vi "Uruchomienie.vi"() -> ()   [LabVIEW 2015]
uses:
  Typedefs/Analiza.ctl
  Typedefs/dane.ctl
  Typedefs/mqttinputs.ctl
  Libraries/MQTT.lvlibp
panel:
  in  "Cisnienie 2":T1 {"P" format="%#.1f"}
  in  "SKSVdial":T2 {"SV" format="%#.1f"; "SK" format="%#.1f"}
  out "value":i32 format="%.0b"
  in  "Start":bool
  out "Zapisane":bool
  in  "Do Bazy":bool
  out "Opis":string
  out "Tacho":dbl format="%#.0f"
  out "Moc Zamowiona":dbl
  out "Typ Palnika":string
  out "Typ Wymiennika":string
  out "SNW":string
  out "SNP":string
  out "cisnienieOK":bool
  in  "Cisnienie":bool
  in  "Analiza":T3 {"I" format="%#.0f"; "CO2" format="%#.1f"; "CO" format="%#.0f"; "O2" format="%#.1f"}
  out "SKSVOK":bool
  in  "SKSV":bool
  out "AnalizaMinKlientOK":bool
  out "AnalizaMaxKlientOK":bool
  out "AnalizaMinOK":bool
  out "AnalizaMaxOK":bool
  in  "AnalizaMinKlient":bool
  in  "AnalizaMaxKlient":bool
  in  "AnalizaMin":bool
  in  "AnalizaMax":bool
  in  "BtnMaxLufa":bool
  in  "BtnMin":bool
  in  "PWMMin":dbl=15.0
  in  "BtnMax Klient":bool
  in  "PWM Max Klient":dbl=90.0
  in  "Kas":bool
  out "Awaria":bool
  out "PWM":dbl
  in  "BtnMax":bool
  in  "PWM Max":dbl=100.0
  in  "BtnMin Klient":bool
  in  "PWMMinKlient":dbl=15.0
  in  "BtnStart":bool
  out "MOC":dbl format="%#_1g"
  in  "Uruchamia:":u16(ring) items=["------", "RADZIWON TOMASZ", "RADZIWON MICHAŁ", "HARBANOWICZ FRANCISZEK", "JANUSZKIEWICZ JAKUB", "PIOTROWSKI DAMIAN", "WISZNIEWSKI JERZY", "BOHM ŁUKASZ"]
  in  "Temat":u16(ring) items=["------", "197-B", "2534-A"]
  in  "PWMStart":dbl=25.0
  in  "Nawiew_f":dbl=7.0
  in  "Nawiew":bool
  out "GAZ":bool
  in  "Zaplon":bool
  # "Hz"
  # "kW"
  # "21-24: 25%\npozostale 45%"
  # "%"
  # "%"
  # "Hz"
  # "%"
  # "%"
  # "%"
  # "%"
  # "Pa"
  # "mm"
  # "mm"
  # "Pmax 4%-5%\nPmin 3%-6.5%"
  # "%"
  # "%"
  # "ppm"
  # "<100ppm"
  # "uA"
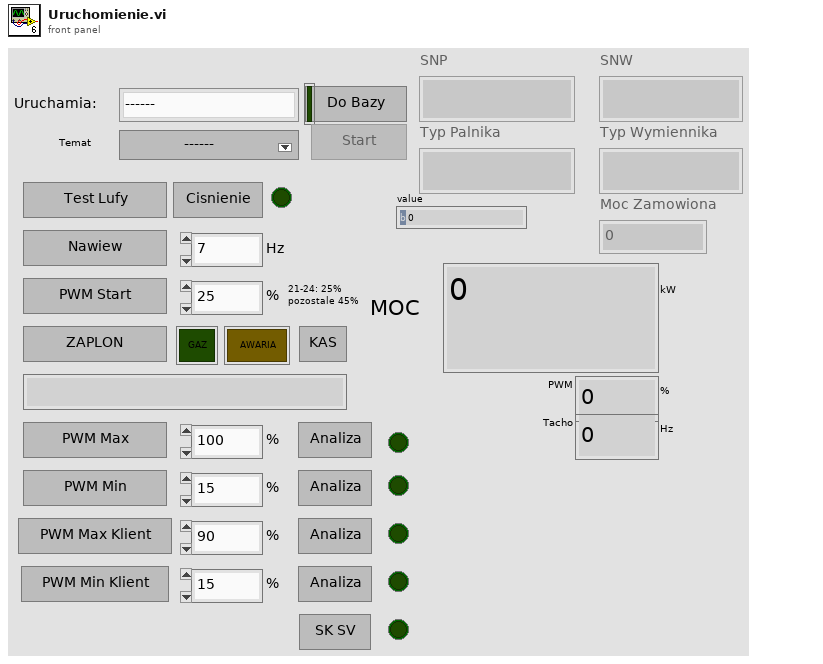
[diagram p1: front panel]
types:
  T1 = cluster{"P":dbl, "OK Button":bool, "Cancel Button":bool}
  T2 = cluster{"SK":dbl, "OK Button":bool, "Cancel Button":bool, "SV":dbl}
  T3 = typedef "Analiza.ctl" = cluster{"O2":dbl, "CO":dbl, "OK Button":bool, "Cancel Button":bool, "CO2":dbl, "I":dbl}
  T4 = typedef "MQTT.lvlibp/Broadcast Events--cluster.ctl" = cluster{"Module Did Init":refnum<user-event>, "Status Updated":refnum<user-event>, "Error Reported":refnum<user-event>, "Module Did Stop":refnum<user-event>, "Update Module Execution Status":refnum<user-event>, "Message":refnum<user-event>}
  T5 = enum8{"Enabled", "Disabled", "Disabled and Grayed Out"}
  T6 = enum32{"invalid app kind", "Development System", "Run Time System", "Student Edition", "Embedded LabVIEW", "Evaluation", "Custom"}
  T7 = typedef "dane.ctl" = cluster{"P":cluster{"max":dbl, "min":dbl, "klientmax":dbl, "klientmin":dbl}, "CO":cluster{"max":dbl, "min":dbl, "klientmax":dbl, "klientmin":dbl}, "CO2":cluster{"max":dbl, "min":dbl, "klientmax":dbl, "klientmin":dbl}, "O2":cluster{"max":dbl, "min":dbl, "klientmax":dbl, "klientmin":dbl}, "I":cluster{"max":dbl, "min":dbl, "klientmax":dbl, "klientmin":dbl}, "n":cluster{"max":dbl, "min":dbl, "klientmax":dbl, "klientmin":dbl}, "pwm":cluster{"klientmax":dbl, "klientmin":dbl}, "valve":cluster{"SK":dbl, "SV":dbl}, "pLufa100":dbl, "data":cluster{"Uruchomil":dbl, "Temat":string, "Podtemat":string, "Uwagi":string}}
  T8 = enum32{"Invalid", "Standard", "Closed", "Hidden", "Minimized", "Maximized"}
  T9 = typedef "mqttinputs.ctl" = cluster{"Power":dbl, "PWM":i32, "Tacho":i32, "Gaz":bool, "Awaria":bool, "dP":dbl, "Praca":bool, "DKG":bool}
  T10 = cluster{refnum<vi>[], "Core":cluster{"Current VI Reference":refnum<vi>, "Close Panel on Exit?":bool}, "controls":refnum<vi>[], "Kto-Lista":string[], "Kto-Lista-Num":i32[], "Kto":u8, "Tematy-Lista":string[], "TematyDane":string[][], "Temat":string, "Data":T7, "PWM":cluster{" start":i32, "min":i32, "max":i32, "moc":i32, "min klient":i32, "max klient":i32}, "CurrentPWM":i32, "broadcasts":variant, "Subscriptions":variant, "Inputs":T9, "Analiza":string}
  T11 = cluster{" start":i32, "min":i32, "max":i32, "moc":i32, "min klient":i32, "max klient":i32}
  T12 = cluster{"Current VI Reference":refnum<vi>, "Close Panel on Exit?":bool}
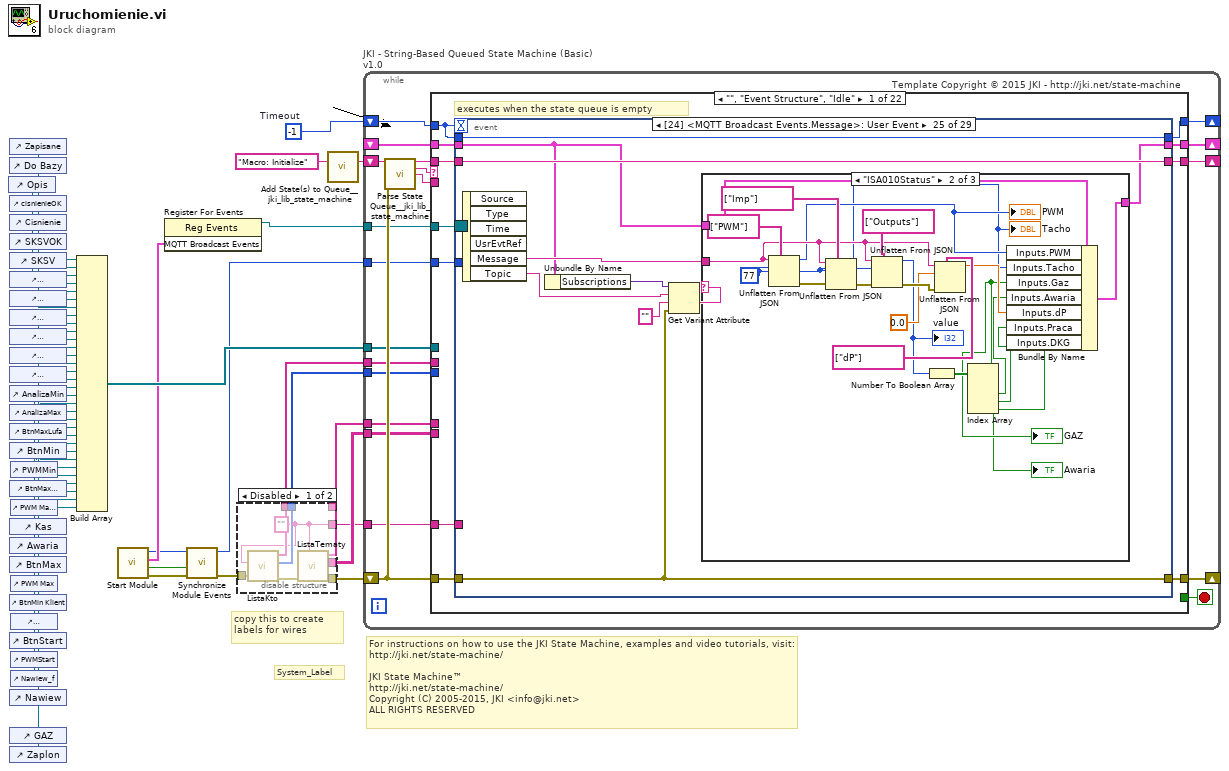
[diagram p0: block diagram]
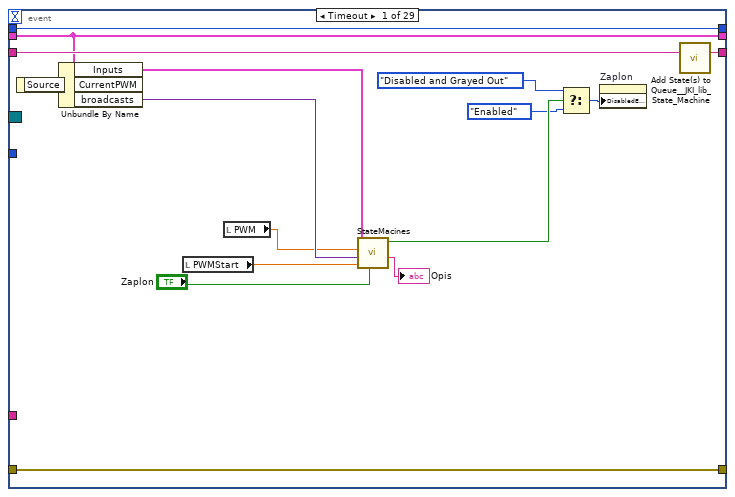
[diagram p3: hidden frame]
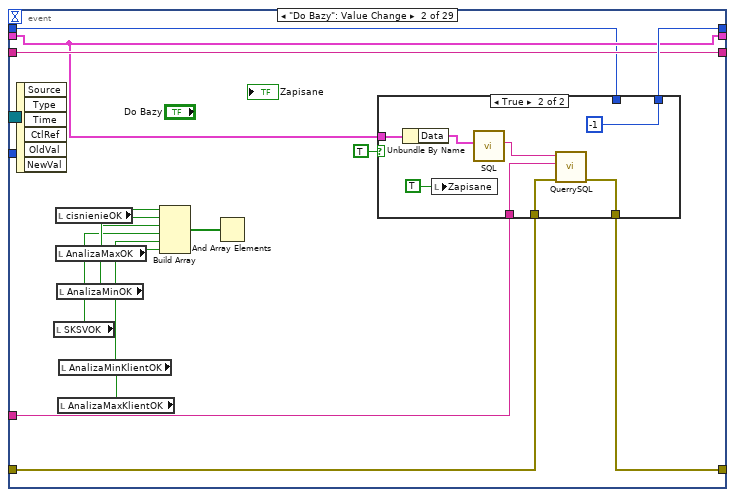
[diagram p4: hidden frame]
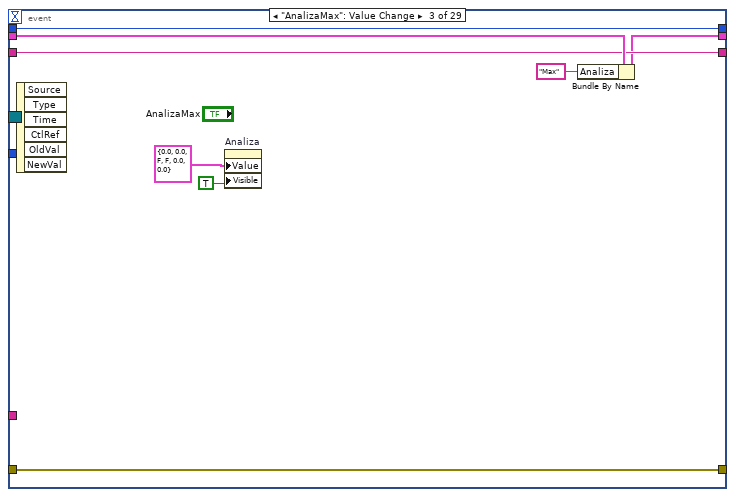
[diagram p6: hidden frame]
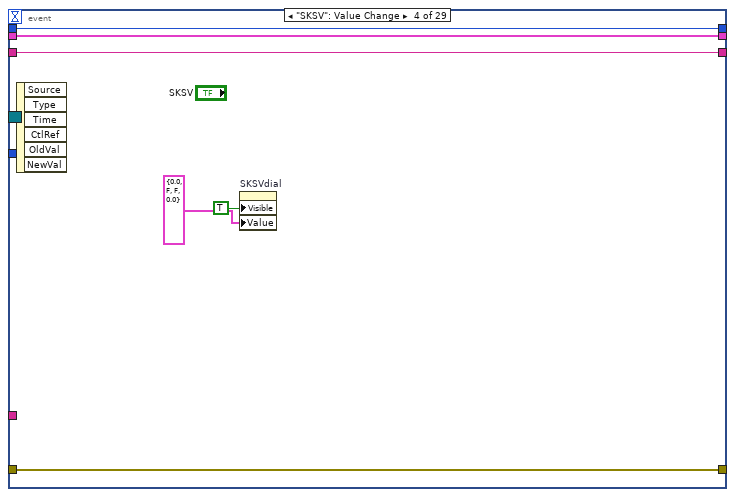
[diagram p7: hidden frame]
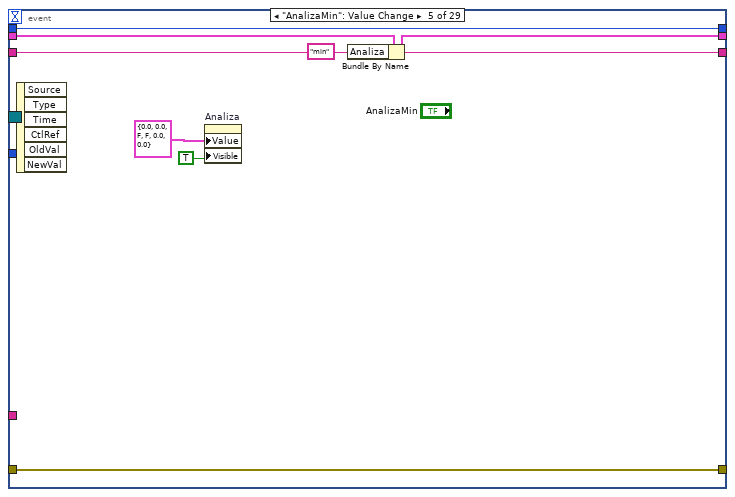
[diagram p8: hidden frame]
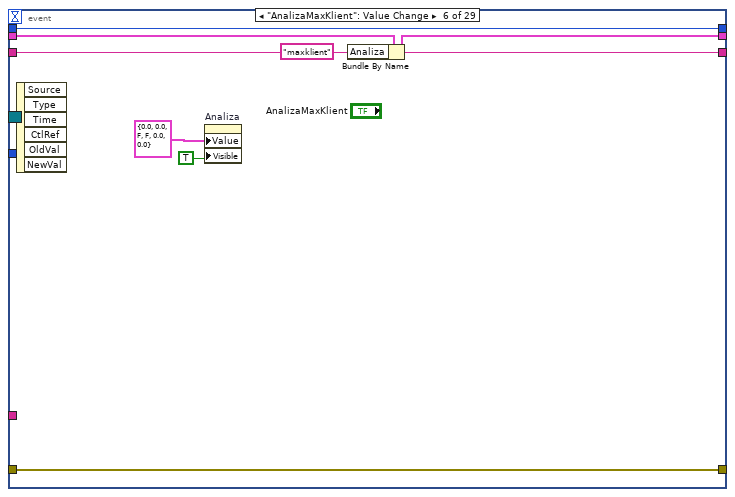
[diagram p9: hidden frame]
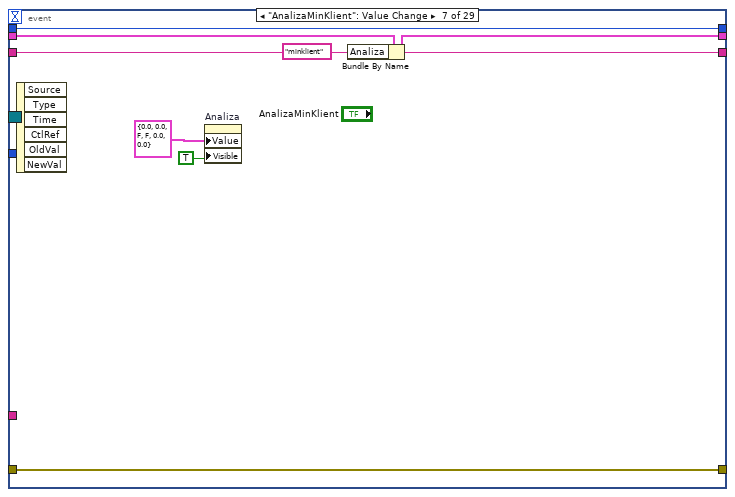
[diagram p10: hidden frame]
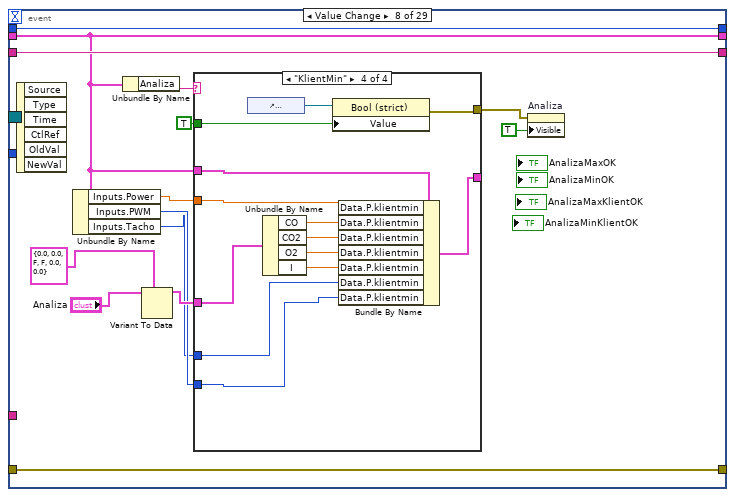
[diagram p11: hidden frame]
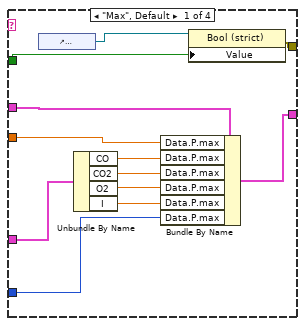
[diagram p12: hidden frame]
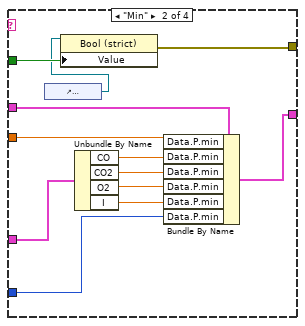
[diagram p13: hidden frame]
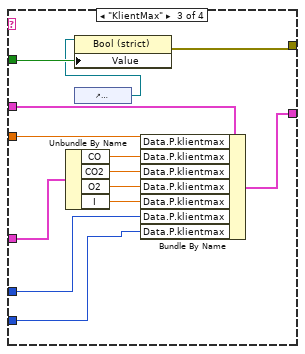
[diagram p14: hidden frame]
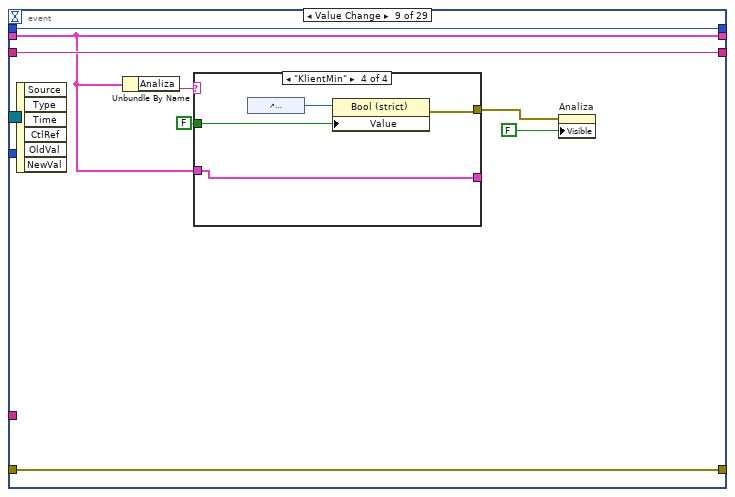
[diagram p15: hidden frame]
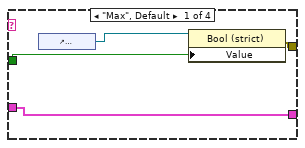
[diagram p16: hidden frame]
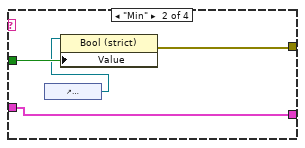
[diagram p17: hidden frame]
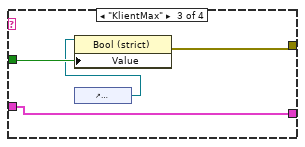
[diagram p18: hidden frame]
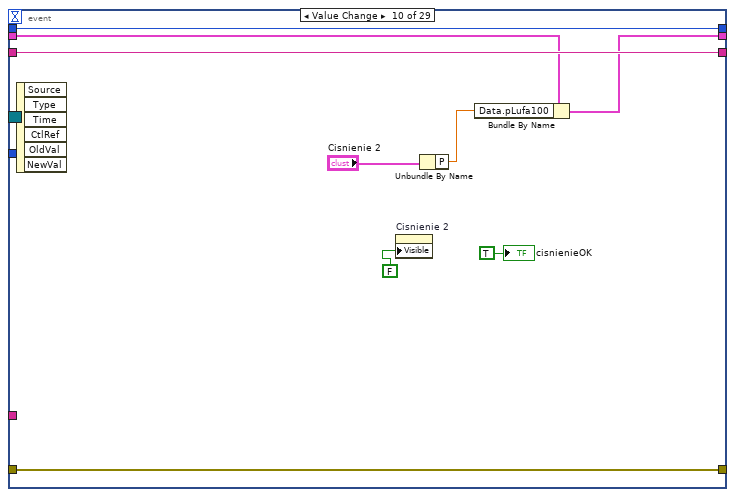
[diagram p19: hidden frame]
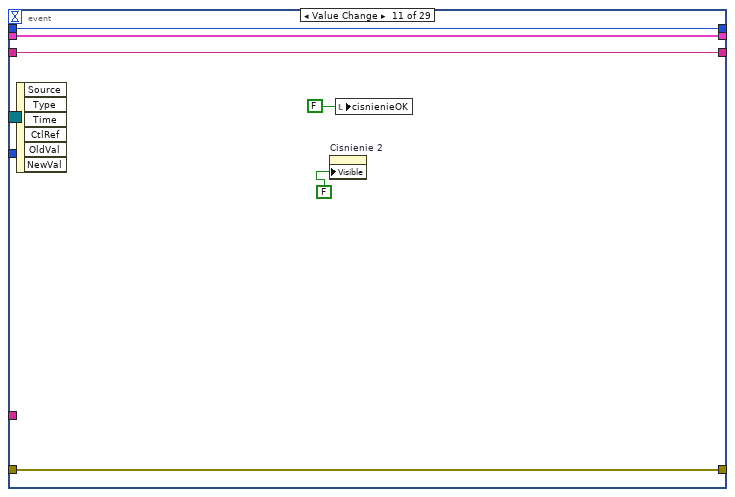
[diagram p20: hidden frame]
diagram:
  w2 = -1  # Timeout
  # "For instructions on how to use the JKI State Machine, examples and video tutorials, visit:\nhttp://jki.net/state-machine/\n\nJKI State Machine™\nhttp://jki.net/state-machine/\nCopyright (C) 2005-2015, JKI <info@jki.net>\nALL RIGHTS RESERVED"
  # "copy this to create labels for wires"
  # "System_Label"
  n1 = control-ref of="Opis"() -> (w47:refnum<vi>)
  n2 = control-ref of="Zapisane"() -> (w49:refnum<vi>)
  n3 = control-ref of="Do Bazy"() -> (w48:refnum<vi>)
  n4 = control-ref of="cisnienieOK"() -> (w46:refnum<vi>)
  n5 = control-ref of="Cisnienie"() -> (w45:refnum<vi>)
  n6 = control-ref of="SKSVOK"() -> (w44:refnum<vi>)
  n7 = control-ref of="SKSV"() -> (w43:refnum<vi>)
  n8 = control-ref of="AnalizaMinKlientOK"() -> (w42:refnum<vi>)
  n9 = control-ref of="AnalizaMaxKlientOK"() -> (w41:refnum<vi>)
  n10 = control-ref of="AnalizaMinOK"() -> (w40:refnum<vi>)
  n11 = control-ref of="AnalizaMaxOK"() -> (w39:refnum<vi>)
  n12 = control-ref of="AnalizaMinKlient"() -> (w38:refnum<vi>)
  n13 = control-ref of="AnalizaMaxKlient"() -> (w37:refnum<vi>)
  n14 = control-ref of="AnalizaMin"() -> (w36:refnum<vi>)
  n15 = control-ref of="AnalizaMax"() -> (w35:refnum<vi>)
  n16 = control-ref of="BtnMaxLufa"() -> (w34:refnum<vi>)
  n17 = control-ref of="BtnMin"() -> (w33:refnum<vi>)
  n18 = control-ref of="BtnMax Klient"() -> (w31:refnum<vi>)
  n19 = control-ref of="Kas"() -> (w29:refnum<vi>)
  n20 = control-ref of="Awaria"() -> (w28:refnum<vi>)
  n21 = control-ref of="BtnMax"() -> (w27:refnum<vi>)
  n22 = control-ref of="BtnMin Klient"() -> (w25:refnum<vi>)
  n23 = control-ref of="BtnStart"() -> (w23:refnum<vi>)
  n24 = control-ref of="Nawiew"() -> (w20:refnum<vi>)
  n25 = control-ref of="GAZ"() -> (w19:refnum<vi>)
  n26 = control-ref of="Zaplon"() -> (w18:refnum<vi>)
  n27 = control-ref of="PWMMin"() -> (w32:refnum<vi>)
  n28 = control-ref of="PWM Max Klient"() -> (w30:refnum<vi>)
  n29 = control-ref of="PWM Max"() -> (w26:refnum<vi>)
  n30 = control-ref of="PWMMinKlient"() -> (w24:refnum<vi>)
  n31 = control-ref of="PWMStart"() -> (w22:refnum<vi>)
  n32 = control-ref of="Nawiew_f"() -> (w21:refnum<vi>)
  n33 = Build Array(w49, w48, w47, w46, w45, w44, w43, w42, w41, w40, w39, w38, w37, w36, w35, w34, w33, w32, w31, w30, w29, w28, w27, w26, w25, w24, w23, w22, w21, w20, w19, w18) -> (w10:refnum<vi>[])
  n34 = call "Start Module.vi"() -> ("error out"=w5:errorcluster, "Wait for Event Sync?"=w6:bool, "MQTT Broadcast Events"=w9:T4, "Module ID"=w8:i32)  [unwired: 8 in]
  n35 = register-events(w9) -> (reference out=w3:refnum<event-registration>)  [unwired: 2 in, 1 out]
  n36 = call "Synchronize Module Events.vi"("error in (no error)"=w5, "Wait for Event Sync?"=w6, "Module ID"=w8) -> ("error out"=w4:errorcluster, "Module ID (dup)"=w7:i32)  [unwired: 7 in]
  n37 = disable-structure shown="Disabled" {
    disable-tunnel: [w57 _] -> w15
    disable-tunnel: [w55 _] -> w14
    disable-tunnel: [w54 _] -> w13
    disable-tunnel: [w53 _] -> w12
    disable-tunnel: [w52 _] -> w11
    disable-tunnel: w4 -> [w51 _]
    disable-tunnel: [w50 _] -> w1
    frame Disabled {
      w50 = "" ("Jsonconfig")
      n38 = call "ListaKto.vi"("error in (no error)"=w51, "Jsonconfig"=w50) -> ("error out"=w56:errorcluster, "Array"=w54:i32[], "Array 2"=w55:string[])  [unwired: 7 in]
      n39 = call "ListaTematy.vi"("Jsonconfig"=w50, "error in (no error)"=w56) -> ("error out"=w57:errorcluster, "data"=w52:string[][], "Array"=w53:string[])  [unwired: 7 in]
    }
    frame Enabled {
    }
  }
  n40 = call <vilib>:"Add State(s) to Queue__jki_lib_state_machine.vi"("State(s) in (\"\")"="Macro: Initialize") -> ("States Out"=w17:string)  [unwired: 14 in]
  n41 = while "JKI - String-Based Queued State Machine (Basic) v1.0" {
    shift-right: [w70] -> _
    shift-left: _ -> [w69]
    shift-right: [w73] -> _
    shift-left: w15 -> [w68]
    shift-right: [w72] -> _
    shift-left: w17 -> [w74]
    tunnel: w14 -> [w67]
    tunnel: w13 -> [w66]
    tunnel: w12 -> [w65]
    tunnel: w11 -> [w64]
    tunnel: w10 -> [w63]
    tunnel: w7 -> [w62]
    tunnel: w3 -> [w61]
    shift-right: [w59] -> _
    shift-left: w2 -> [w60]
    tunnel: w1 -> [w58]
    stop <- w71 stop-if-true
    # "Template Copyright © 2015 JKI - http://jki.net/state-machine"
    n42 = call <vilib>:"Parse State Queue__jki_lib_state_machine.vi"("State Queue"=w74, "Error In (no error)"=w68) -> ("Remaining States"=w76:string, "Current State"=w77:string, "Arguments"=w75:string)  [unwired: 11 in]
    n43 = case shown="\"\", \"Event Structure\", \"Idle\"" w77 {
      selector: w77 -> [_ _ w527 _ _ _ _ _ _ _ _ _ _ _ _ _ _ _ _ _ _ _]
      tunnel: w76 -> [w88 w525 w531 w551 w558 w569 w574 w603 w610 w615 w626 w631 w636 w652 w661 w673 w700 w706 w717 w722 w727 w732]
      tunnel: w75 -> [_ _ _ _ _ _ _ _ _ _ _ _ _ w637 w656 w667 _ _ _ _ _ _]
      tunnel: w69 -> [w86 w522 w529 w542 w555 w567 w571 _ w605 w612 w620 w628 w633 w648 w659 w669 w697 w703 w714 w719 w724 w729]
      tunnel: [w85 w523 w533 w548 errorcluster {"status"=FALSE, "code"=0, "source"=""} ("error out") w560 w572 w600 w606 w613 w622 w629 w634 w650 w657 w670 w698 w704 w715 w720 w725 w730] -> w73
      tunnel: w68 -> [w84 w523 w532 w548 w554 w561 w572 w600 w607 w613 w623 w629 w634 w650 w658 w671 w698 w704 w715 w720 w725 w730]
      tunnel: [w87 w524 w530 w550 w557 w568 w573 w602 w609 w614 w625 w630 w635 w651 w660 w672 w699 w705 w716 w721 w726 w731] -> w72
      tunnel: [_ _ _ _ _ TRUE _ _ _ _ _ _ _ _ _ _ _ _ _ _ _ _] -> w71
      tunnel: [w83 w522 w529 w549 w555 w567 w571 w601 w605 w612 w619 w628 w633 w648 w659 w669 w697 w703 w714 w719 w724 w729] -> w70
      tunnel: w60 -> [w80 w521 w526 w539 w552 w559 w570 w576 w604 w611 w616 w627 w632 w638 w655 w666 w696 w701 w707 w718 w723 w728]
      tunnel: w67 -> [_ _ _ _ _ _ _ w587 _ _ _ _ _ _ _ _ _ _ _ _ _ _]
      tunnel: w66 -> [_ _ _ _ _ _ _ w586 _ _ _ _ _ _ _ _ _ _ _ _ _ _]
      tunnel: w65 -> [_ _ _ _ _ _ _ w585 _ _ _ _ _ _ _ _ _ _ _ _ _ _]
      tunnel: w64 -> [_ _ _ _ _ _ _ w584 _ _ _ _ _ _ _ _ _ _ _ _ _ _]
      tunnel: w63 -> [_ _ _ w538 _ _ _ w582 _ _ _ _ _ _ _ _ _ _ _ _ _ _]
      tunnel: w62 -> [w82 _ _ _ _ w562 _ _ _ _ w624 _ _ _ _ _ _ _ _ _ _ _]
      tunnel: w61 -> [w81 _ _ _ _ w565 _ _ _ _ _ _ _ _ _ _ _ _ _ _ _ _]
      tunnel: [w79 w521 w526 w539 w552 w559 w570 w576 w604 w611 w616 w627 w632 w638 w655 w666 w696 w701 w707 w718 w723 w728] -> w59
      tunnel: w58 -> [w78 _ _ _ _ _ _ _ _ _ _ _ _ _ _ _ _ _ _ _ _ _]
      frame "", "Event Structure", "Idle" {
        # "executes when the state queue is empty"
        n44 = event shown="[24] <MQTT Broadcast Events.Message>: User Event" {
          selector: w81 -> [_ _ _ _ _ _ _ _ _ _ _ _ _ _ _ _ _ _ _ _ _ _ _ _ _ _ _ _ _]
          dyn-events: _ -> [_ _ _ _ _ _ _ _ _ _ _ _ _ _ _ _ _ _ _ _ _ _ _ _ _ _ _ _ _]
          timeout: w80 -> [_ _ _ _ _ _ _ _ _ _ _ _ _ _ _ _ _ _ _ _ _ _ _ _ _ _ _ _ _]
          tunnel: w88 -> [w103 w117 w133 w142 w150 w158 w166 w180 w238 w263 w269 w279 w285 w291 w311 w325 w334 w359 w371 w383 w395 w407 w419 w439 w449 w482 w488 w510 w520]
          tunnel: [w102 w117 w133 w142 w150 w158 w166 w180 w238 w263 w269 w279 w285 w291 w311 w325 w334 w359 w371 w383 w395 w407 w419 w439 w449 w482 w489 w510 w519] -> w87
          tunnel: w86 -> [w96 w116 w134 w140 w148 w156 w164 w170 w233 w259 w267 w273 w283 w289 w309 w323 w332 w357 w369 w381 w393 w405 w417 w437 w442 w480 w490 w508 w517]
          tunnel: [w101 w113 w135 w141 w149 w157 w165 w179 w237 w262 w268 w278 w284 w290 w297 w317 w329 w354 w366 w378 w390 w402 w414 w421 w444 w478 w486 w493 w518] -> w85
          tunnel: w84 -> [w101 w114 w135 w141 w149 w157 w165 w179 w237 w262 w268 w278 w284 w290 w298 w316 w328 w353 w365 w377 w389 w401 w413 w432 w444 w478 w486 w493 w518]
          tunnel: [w96 w116 w132 w140 w144 w152 w160 w170 w233 w258 w267 w272 w283 w289 w309 w323 w332 w357 w369 w381 w393 w405 w417 w437 w441 w479 w490 w509 w517] -> w83
          tunnel: w82 -> [_ _ _ _ _ _ _ _ _ _ _ _ _ _ w301 w319 w330 w355 w367 w379 w391 w403 w415 w423 _ _ _ _ _]
          tunnel: w80 -> [w93 w104 w136 w139 w147 w155 w163 w178 w236 w261 w266 w277 w282 w288 w310 w324 w333 w358 w370 w382 w394 w406 w418 w438 w440 w477 _ w491 w514]
          tunnel: [w93 w118 w136 w139 w147 w155 w163 w178 w236 w261 w266 w277 w282 w288 w310 w324 w333 w358 w370 w382 w394 w406 w418 w438 w440 w477 500 ("Timeout") w491 w514] -> w79
          tunnel: w78 -> [_ w115 _ _ _ _ _ _ _ _ _ _ _ _ _ _ _ _ _ _ _ _ _ _ _ _ _ _ _]
          event Timeout {
            n45 = event-data() -> ()  [unwired: 1 in, 1 out]
            n46 = Unbundle By Name(w96) -> ("Inputs"=w95:T9, "broadcasts"=w94:variant)  [unwired: 1 out]
            n47 = local read "PWMStart"() -> (w92:dbl)
            n48 = local read "PWM"() -> (w89:dbl)
            n49 = call "StateMacines.vi"("Operate"="Zaplon", "PWMStart"=w92, "broadcasts"=w94, "CurrentPWM"=w89, "Inputs"=w95) -> ("Opis"=→"Opis":string, "DisableStartBtn"=w100:bool)  [unwired: 4 in, 1 out]
            n50 = Select(t=T5."Disabled and Grayed Out" ("Disabled"), s=w100, f=T5."Enabled" ("Disabled")) -> (s? t:f=w97:T5)
            n51 = property on="Zaplon" class="Bool (strict)"("DisabledEnum"=w97) -> ()  [unwired: 2 in, 2 out]
            n52 = call <vilib>:"Add State(s) to Queue__JKI_lib_State_Machine.vi"("State(s) in (\"\")"=w103) -> ("States Out"=w102:string)  [unwired: 14 in]
          }
          event "Do Bazy": Value Change {
            n53 = event-data() -> ()  [unwired: 1 in, 6 out]
            n54 = local read "SKSVOK"() -> (w109:bool)
            n55 = local read "cisnienieOK"() -> (w112:bool)
            n56 = local read "AnalizaMaxOK"() -> (w111:bool)
            n57 = local read "AnalizaMinOK"() -> (w110:bool)
            n58 = local read "AnalizaMaxKlientOK"() -> (w107:bool)
            n59 = local read "AnalizaMinKlientOK"() -> (w108:bool)
            n60 = Build Array(w112, w111, w110, w109, w108, w107) -> (w106:bool[])
            n61 = And Array Elements(Boolean array=w106) -> ()  [unwired: 1 out]
            n62 = case shown="True" TRUE {
              tunnel: [w119 -1 ("Timeout")] -> w118
              tunnel: w116 -> [_ w127]
              tunnel: w115 -> [_ w124]
              tunnel: w114 -> [w120 w123]
              tunnel: [w120 w122] -> w113
              tunnel: w104 -> [w119 _]
              frame False {
              }
              frame True {
                n63 = Unbundle By Name(w127) -> ("Data"=w126:T7)
                n64 = local write "Zapisane"(TRUE ("Zapisane")) -> ()
                n65 = call "SQL.vi"("Data"=w126) -> ("SQL querry"=w125:string)  [unwired: 9 in, 1 out]
                n66 = call "QuerrySQL.vi"("error in (no error)"=w123, "Jsonconfig"=w124, "String"=w125) -> ("error out"=w122:errorcluster)  [unwired: 7 in, 1 out]
              }
            }
          }
          event "AnalizaMax": Value Change {
            n67 = event-data() -> ()  [unwired: 1 in, 6 out]
            n68 = property on="Analiza" class="Clust"("Value"=T3 {"O2"=0.0, "CO"=0.0, "OK Button"=FALSE, "Cancel Button"=FALSE, "CO2"=0.0, "I"=0.0} ("Analiza"), "Visible"=TRUE) -> ()  [unwired: 2 in, 2 out]
            n69 = Bundle By Name(cluster=w134, "Analiza"="Max") -> (w132:T10)
          }
          event "SKSV": Value Change {
            n70 = event-data() -> ()  [unwired: 1 in, 6 out]
            n71 = property on="SKSVdial" class="Clust"("Visible"=TRUE, "Value"=T2 {"SK"=0.0, "OK Button"=FALSE, "Cancel Button"=FALSE, "SV"=0.0} ("SKSV")) -> ()  [unwired: 2 in, 2 out]
          }
          event "AnalizaMin": Value Change {
            n72 = event-data() -> ()  [unwired: 1 in, 6 out]
            n73 = property on="Analiza" class="Clust"("Value"=T3 {"O2"=0.0, "CO"=0.0, "OK Button"=FALSE, "Cancel Button"=FALSE, "CO2"=0.0, "I"=0.0} ("Analiza"), "Visible"=TRUE) -> ()  [unwired: 2 in, 2 out]
            n74 = Bundle By Name(cluster=w148, "Analiza"="min") -> (w144:T10)
          }
          event "AnalizaMaxKlient": Value Change {
            n75 = event-data() -> ()  [unwired: 1 in, 6 out]
            n76 = property on="Analiza" class="Clust"("Value"=T3 {"O2"=0.0, "CO"=0.0, "OK Button"=FALSE, "Cancel Button"=FALSE, "CO2"=0.0, "I"=0.0} ("Analiza"), "Visible"=TRUE) -> ()  [unwired: 2 in, 2 out]
            n77 = Bundle By Name(cluster=w156, "Analiza"="maxklient") -> (w152:T10)
          }
          event "AnalizaMinKlient": Value Change {
            n78 = event-data() -> ()  [unwired: 1 in, 6 out]
            n79 = property on="Analiza" class="Clust"("Value"=T3 {"O2"=0.0, "CO"=0.0, "OK Button"=FALSE, "Cancel Button"=FALSE, "CO2"=0.0, "I"=0.0} ("Analiza"), "Visible"=TRUE) -> ()  [unwired: 2 in, 2 out]
            n80 = Bundle By Name(cluster=w164, "Analiza"="minklient") -> (w160:T10)
          }
          event Value Change {
            n81 = event-data() -> ()  [unwired: 1 in, 6 out]
            n82 = Unbundle By Name(w170) -> ("Inputs.Power"=w169:dbl, "Inputs.PWM"=w168:i32, "Inputs.Tacho"=w167:i32)
            n83 = Unbundle By Name(w170) -> ("Analiza"=w174:string)
            n84 = Variant To Data(type=T3 {"O2"=0.0, "CO"=0.0, "OK Button"=FALSE, "Cancel Button"=FALSE, "CO2"=0.0, "I"=0.0} ("Analiza"), Variant="Analiza") -> (data=w176:T3)  [unwired: 1 in, 1 out]
            n85 = case shown="\"KlientMin\"" w174 {
              tunnel: TRUE ("AnalizaMinOK") -> [w192 w204 w217 w230]
              tunnel: [w191 w203 w216 w229] -> w173
              tunnel: [w186 w198 w214 w223] -> _
              tunnel: w170 -> [w185 w197 w215 w224]
              tunnel: w176 -> [w184 w195 w213 w221]
              tunnel: w169 -> [w183 w196 w208 w222]
              tunnel: w167 -> [w182 w194 w207 w220]
              tunnel: w168 -> [_ _ w206 w219]
              frame "Max", Default {
                n86 = control-ref of="AnalizaMaxOK"() -> (w181:refnum<vi>)
                n87 = Unbundle By Name(w184) -> ("CO"=w190:dbl, "CO2"=w189:dbl, "O2"=w188:dbl, "I"=w187:dbl)
                n88 = Bundle By Name(cluster=w185, "Data.P.max"=w183, "Data.P.max"=w190, "Data.P.max"=w189, "Data.P.max"=w188, "Data.P.max"=w187, "Data.P.max"=w182) -> (w186:T10)
                n89 = property on="Property Node" class="Bool (strict)"(reference=w181, "Value"=w192) -> (error out=w191:errorcluster)  [unwired: 1 in, 1 out]
              }
              frame "Min" {
                n90 = control-ref of="AnalizaMinOK"() -> (w193:refnum<vi>)
                n91 = property on="Property Node" class="Bool (strict)"(reference=w193, "Value"=w204) -> (error out=w203:errorcluster)  [unwired: 1 in, 1 out]
                n92 = Unbundle By Name(w195) -> ("CO"=w202:dbl, "CO2"=w201:dbl, "O2"=w200:dbl, "I"=w199:dbl)
                n93 = Bundle By Name(cluster=w197, "Data.P.min"=w196, "Data.P.min"=w202, "Data.P.min"=w201, "Data.P.min"=w200, "Data.P.min"=w199, "Data.P.min"=w194) -> (w198:T10)
              }
              frame "KlientMax" {
                n94 = Unbundle By Name(w213) -> ("CO"=w209:dbl, "CO2"=w210:dbl, "O2"=w211:dbl, "I"=w212:dbl)
                n95 = control-ref of="AnalizaMaxKlientOK"() -> (w205:refnum<vi>)
                n96 = property on="Property Node" class="Bool (strict)"(reference=w205, "Value"=w217) -> (error out=w216:errorcluster)  [unwired: 1 in, 1 out]
                n97 = Bundle By Name(cluster=w215, "Data.P.klientmax"=w208, "Data.P.klientmax"=w209, "Data.P.klientmax"=w210, "Data.P.klientmax"=w211, "Data.P.klientmax"=w212, "Data.P.klientmax"=w207, "Data.P.klientmax"=w206) -> (w214:T10)
              }
              frame "KlientMin" {
                n98 = control-ref of="AnalizaMinKlientOK"() -> (w218:refnum<vi>)
                n99 = Unbundle By Name(w221) -> ("CO"=w228:dbl, "CO2"=w227:dbl, "O2"=w226:dbl, "I"=w225:dbl)
                n100 = property on="Property Node" class="Bool (strict)"(reference=w218, "Value"=w230) -> (error out=w229:errorcluster)  [unwired: 1 in, 1 out]
                n101 = Bundle By Name(cluster=w224, "Data.P.klientmin"=w222, "Data.P.klientmin"=w228, "Data.P.klientmin"=w227, "Data.P.klientmin"=w226, "Data.P.klientmin"=w225, "Data.P.klientmin"=w220, "Data.P.klientmin"=w219) -> (w223:T10)
              }
            }
            n102 = property on="Analiza" class="Clust"(error in=w173, "Visible"=TRUE) -> ()  [unwired: 1 in, 2 out]
          }
          event Value Change {
            n103 = event-data() -> ()  [unwired: 1 in, 6 out]
            n104 = Unbundle By Name(w233) -> ("Analiza"=w235:string)
            n105 = case shown="\"KlientMin\"" w235 {
              tunnel: FALSE ("AnalizaMinOK") -> [w242 w246 w250 w254]
              tunnel: [w241 w245 w249 w253] -> w232
              tunnel: [w240 w244 w248 w252] -> _
              tunnel: w233 -> [w240 w244 w248 w252]
              frame "Max", Default {
                n106 = control-ref of="AnalizaMaxOK"() -> (w239:refnum<vi>)
                n107 = property on="Property Node" class="Bool (strict)"(reference=w239, "Value"=w242) -> (error out=w241:errorcluster)  [unwired: 1 in, 1 out]
              }
              frame "Min" {
                n108 = control-ref of="AnalizaMinOK"() -> (w243:refnum<vi>)
                n109 = property on="Property Node" class="Bool (strict)"(reference=w243, "Value"=w246) -> (error out=w245:errorcluster)  [unwired: 1 in, 1 out]
              }
              frame "KlientMax" {
                n110 = control-ref of="AnalizaMaxKlientOK"() -> (w247:refnum<vi>)
                n111 = property on="Property Node" class="Bool (strict)"(reference=w247, "Value"=w250) -> (error out=w249:errorcluster)  [unwired: 1 in, 1 out]
              }
              frame "KlientMin" {
                n112 = control-ref of="AnalizaMinKlientOK"() -> (w251:refnum<vi>)
                n113 = property on="Property Node" class="Bool (strict)"(reference=w251, "Value"=w254) -> (error out=w253:errorcluster)  [unwired: 1 in, 1 out]
              }
            }
            n114 = property on="Analiza" class="Clust"(error in=w232, "Visible"=FALSE) -> ()  [unwired: 1 in, 2 out]
          }
          event "Cisnienie 2.OK Button": Value Change {
            n115 = event-data() -> ()  [unwired: 1 in, 6 out]
            n116 = property on="Cisnienie 2" class="Clust"("Visible"=FALSE) -> ()  [unwired: 2 in, 2 out]
            n117 = Unbundle By Name("Cisnienie 2") -> ("P"=w260:dbl)
            n118 = Bundle By Name(cluster=w259, "Data.pLufa100"=w260) -> (w258:T10)
            "cisnienieOK" <- TRUE ("cisnienieOK")
          }
          event "Cisnienie 2.Cancel Button": Value Change {
            n119 = event-data() -> ()  [unwired: 1 in, 6 out]
            n120 = property on="Cisnienie 2" class="Clust"("Visible"=FALSE) -> ()  [unwired: 2 in, 2 out]
            n121 = local write "cisnienieOK"(FALSE ("cisnienieOK")) -> ()
          }
          event "SKSVdial.OK Button": Value Change {
            n122 = event-data() -> ()  [unwired: 1 in, 6 out]
            n123 = property on="SKSVdial" class="Clust"("Visible"=FALSE) -> ()  [unwired: 2 in, 2 out]
            n124 = Unbundle By Name("SKSVdial") -> ("SK"=w275:dbl, "SV"=w274:dbl)
            n125 = Bundle By Name(cluster=w273, "Data.valve.SK"=w275, "Data.valve.SV"=w274) -> (w272:T10)
            "SKSVOK" <- TRUE ("SKSVOK")
          }
          event "SKSVdial.Cancel Button": Value Change {
            n126 = event-data() -> ()  [unwired: 1 in, 6 out]
            n127 = property on="SKSVdial" class="Clust"("Visible"=FALSE) -> ()  [unwired: 2 in, 2 out]
            n128 = local write "SKSVOK"(FALSE ("SKSVOK")) -> ()
          }
          event "Cisnienie": Value Change {
            n129 = event-data() -> ()  [unwired: 1 in, 6 out]
            n130 = property on="Cisnienie 2" class="Clust"("Value"=T1 {"P"=0.0, "OK Button"=FALSE, "Cancel Button"=FALSE} ("Cisnienie 2"), "Visible"=TRUE) -> ()  [unwired: 2 in, 2 out]
          }
          event "Nawiew": Value Change {
            w304 = "InverterDrive"
            w307 = "InverterEngage"
            n131 = event-data() -> ()  [unwired: 1 in, 6 out]
            n132 = case shown="False" "Nawiew" {
              tunnel: [0.0 ("Nawiew_f") w313] -> w296
              frame False {
              }
              frame True {
                n133 = local read "Nawiew_f"() -> (w313:dbl)
              }
            }
            n134 = Unbundle By Name(w309) -> ("broadcasts"=w308:variant)
            n135 = Get Variant Attribute(Variant=w308, name=w307, default value (empty Variant)=w307, error in=w298) -> (duplicate Variant=w305:variant, value=w302:string, error out=w306:errorcluster)  [unwired: 1 out]
            n136 = Boolean To (0,1)(Boolean="Nawiew") -> (0, 1=w293:i16)
            n137 = Format Into String(w293) -> (resulting string=w292:string)  [unwired: 3 in, 1 out]
            n138 = Format Into String(w296) -> (resulting string=w295:string)  [unwired: 3 in, 1 out]
            n139 = Get Variant Attribute(Variant=w305, name=w304, default value (empty Variant)=w304, error in=w306) -> (value=w303:string, error out=w300:errorcluster)  [unwired: 2 out]
            n140 = call "Publish.vi"("error in (no error)"=w300, "Payload"=w295, "Topic"=w303, "Module ID"=w301) -> ("error out"=w299:errorcluster)  [unwired: 7 in]
            n141 = call "Publish.vi"("error in (no error)"=w299, "Payload"=w292, "Topic"=w302, "Module ID"=w301) -> ("error out"=w297:errorcluster)  [unwired: 7 in]
          }
          event "Nawiew_f": Value Change {
            w321 = "InverterDrive"
            n142 = event-data() -> ()  [unwired: 1 in, 6 out]
            n143 = Unbundle By Name(w323) -> ("broadcasts"=w322:variant)
            n144 = Format Into String("Nawiew_f") -> (resulting string=w315:string)  [unwired: 3 in, 1 out]
            n145 = Get Variant Attribute(Variant=w322, name=w321, default value (empty Variant)=w321, error in=w316) -> (value=w320:string, error out=w318:errorcluster)  [unwired: 2 out]
            n146 = call "Publish.vi"("error in (no error)"=w318, "Payload"=w315, "Topic"=w320, "Module ID"=w319) -> ("error out"=w317:errorcluster)  [unwired: 7 in]
          }
          event "PWM Max", "PWMMin", "PWM Max Klient", "PWMMinKlient", "PWMStart": Value Change {
            n147 = event-data() -> ("NewVal"=w327:dbl)  [unwired: 1 in, 5 out]
            n148 = Unbundle By Name(w332) -> ("Inputs.Praca"=w326:bool, "broadcasts"=w331:variant)
            n149 = case shown="False" w326 {
              tunnel: w331 -> [_ w344]
              tunnel: w330 -> [_ w341]
              tunnel: [w335 w339] -> w329
              tunnel: w328 -> [w335 w338]
              tunnel: w327 -> [_ w336]
              frame False {
              }
              frame True {
                w343 = "ISAPWM"
                n150 = Format Into String(w336) -> (resulting string=w337:string)  [unwired: 3 in, 1 out]
                n151 = Get Variant Attribute(Variant=w344, name=w343, default value (empty Variant)=w343, error in=w338) -> (value=w342:string, error out=w340:errorcluster)  [unwired: 2 out]
                n152 = call "Publish.vi"("error in (no error)"=w340, "Payload"=w337, "Topic"=w342, "Module ID"=w341) -> ("error out"=w339:errorcluster)  [unwired: 7 in]
              }
            }
          }
          event "BtnMaxLufa": Value Change {
            w352 = "ISAPWM"
            n153 = event-data() -> ()  [unwired: 1 in, 6 out]
            n154 = Unbundle By Name(w357) -> ("broadcasts"=w356:variant)
            n155 = Select(t=100, s="BtnMaxLufa", f=0) -> (s? t:f=w345:i32)
            n156 = Format Into String(w345) -> (resulting string=w349:string)  [unwired: 3 in, 1 out]
            n157 = Get Variant Attribute(Variant=w356, name=w352, default value (empty Variant)=w352, error in=w353) -> (value=w351:string, error out=w350:errorcluster)  [unwired: 2 out]
            n158 = call "Publish.vi"("error in (no error)"=w350, "Payload"=w349, "Topic"=w351, "Module ID"=w355) -> ("error out"=w354:errorcluster)  [unwired: 7 in]
          }
          event "BtnMax Klient": Value Change {
            w364 = "ISAPWM"
            n159 = event-data() -> ()  [unwired: 1 in, 6 out]
            n160 = local read "PWM Max Klient"() -> (w360:dbl)
            n161 = Unbundle By Name(w369) -> ("broadcasts"=w368:variant)
            n162 = Format Into String(w360) -> (resulting string=w361:string)  [unwired: 3 in, 1 out]
            n163 = Get Variant Attribute(Variant=w368, name=w364, default value (empty Variant)=w364, error in=w365) -> (value=w363:string, error out=w362:errorcluster)  [unwired: 2 out]
            n164 = call "Publish.vi"("error in (no error)"=w362, "Payload"=w361, "Topic"=w363, "Module ID"=w367) -> ("error out"=w366:errorcluster)  [unwired: 7 in]
          }
          event "BtnMin Klient": Value Change {
            w376 = "ISAPWM"
            n165 = event-data() -> ()  [unwired: 1 in, 6 out]
            n166 = local read "PWMMinKlient"() -> (w372:dbl)
            n167 = Unbundle By Name(w381) -> ("broadcasts"=w380:variant)
            n168 = Format Into String(w372) -> (resulting string=w373:string)  [unwired: 3 in, 1 out]
            n169 = Get Variant Attribute(Variant=w380, name=w376, default value (empty Variant)=w376, error in=w377) -> (value=w375:string, error out=w374:errorcluster)  [unwired: 2 out]
            n170 = call "Publish.vi"("error in (no error)"=w374, "Payload"=w373, "Topic"=w375, "Module ID"=w379) -> ("error out"=w378:errorcluster)  [unwired: 7 in]
          }
          event "BtnMax": Value Change {
            w388 = "ISAPWM"
            n171 = event-data() -> ()  [unwired: 1 in, 6 out]
            n172 = local read "PWM Max"() -> (w384:dbl)
            n173 = Unbundle By Name(w393) -> ("broadcasts"=w392:variant)
            n174 = Format Into String(w384) -> (resulting string=w385:string)  [unwired: 3 in, 1 out]
            n175 = Get Variant Attribute(Variant=w392, name=w388, default value (empty Variant)=w388, error in=w389) -> (value=w387:string, error out=w386:errorcluster)  [unwired: 2 out]
            n176 = call "Publish.vi"("error in (no error)"=w386, "Payload"=w385, "Topic"=w387, "Module ID"=w391) -> ("error out"=w390:errorcluster)  [unwired: 7 in]
          }
          event "BtnMin": Value Change {
            w400 = "ISAPWM"
            n177 = event-data() -> ()  [unwired: 1 in, 6 out]
            n178 = local read "PWMMin"() -> (w396:dbl)
            n179 = Unbundle By Name(w405) -> ("broadcasts"=w404:variant)
            n180 = Format Into String(w396) -> (resulting string=w397:string)  [unwired: 3 in, 1 out]
            n181 = Get Variant Attribute(Variant=w404, name=w400, default value (empty Variant)=w400, error in=w401) -> (value=w399:string, error out=w398:errorcluster)  [unwired: 2 out]
            n182 = call "Publish.vi"("error in (no error)"=w398, "Payload"=w397, "Topic"=w399, "Module ID"=w403) -> ("error out"=w402:errorcluster)  [unwired: 7 in]
          }
          event "BtnStart": Value Change {
            w412 = "ISAPWM"
            n183 = event-data() -> ()  [unwired: 1 in, 6 out]
            n184 = local read "PWMStart"() -> (w408:dbl)
            n185 = Unbundle By Name(w417) -> ("broadcasts"=w416:variant)
            n186 = Format Into String(w408) -> (resulting string=w409:string)  [unwired: 3 in, 1 out]
            n187 = Get Variant Attribute(Variant=w416, name=w412, default value (empty Variant)=w412, error in=w413) -> (value=w411:string, error out=w410:errorcluster)  [unwired: 2 out]
            n188 = call "Publish.vi"("error in (no error)"=w410, "Payload"=w409, "Topic"=w411, "Module ID"=w415) -> ("error out"=w414:errorcluster)  [unwired: 7 in]
          }
          event "Kas": Value Change {
            w426 = "ISAPWM"
            w435 = "ISAKASAWAR"
            n189 = event-data() -> ("NewVal"=w429:bool)  [unwired: 1 in, 5 out]
            n190 = Unbundle By Name(w437) -> ("broadcasts"=w436:variant)
            n191 = local read "PWMStart"() -> (w420:dbl)
            n192 = Boolean To (0,1)(Boolean=w429) -> (0, 1=w430:i16)
            n193 = Format Into String(w430) -> (resulting string=w431:string)  [unwired: 3 in, 1 out]
            n194 = Format Into String(w420) -> (resulting string=w422:string)  [unwired: 3 in, 1 out]
            n195 = Get Variant Attribute(Variant=w436, name=w435, default value (empty Variant)=w435, error in=w432) -> (duplicate Variant=w424:variant, value=w434:string, error out=w433:errorcluster)  [unwired: 1 out]
            n196 = call "Publish.vi"("error in (no error)"=w433, "Payload"=w431, "Topic"=w434, "Module ID"=w423) -> ("error out"=w425:errorcluster)  [unwired: 7 in]
            n197 = Get Variant Attribute(Variant=w424, name=w426, default value (empty Variant)=w426, error in=w425) -> (value=w427:string, error out=w428:errorcluster)  [unwired: 2 out]
            n198 = call "Publish.vi"("error in (no error)"=w428, "Payload"=w422, "Topic"=w427, "Module ID"=w423) -> ("error out"=w421:errorcluster)  [unwired: 7 in]
          }
          event User Event {
            n199 = event-data() -> ("Message"=w443:string, "Topic"=w447:string)  [unwired: 1 in, 4 out]
            n200 = Unbundle By Name(w442) -> ("Subscriptions"=w448:variant)
            n201 = Get Variant Attribute(Variant=w448, name=w447, default value (empty Variant)="" ("Topic"), error in=w444) -> (value=w446:string)  [unwired: 3 out]
            n202 = case shown="\"ISA010Status\"" w446 {
              tunnel: w443 -> [_ w463 w476]
              tunnel: w442 -> [w450 w461 w475]
              tunnel: [w450 w459 w474] -> w441
              frame Default {
              }
              frame "ISA010Status" {
                w467 = 77
                n203 = Unflatten From JSON(path=string[] ["PWM"], JSON string=w463, type and defaults=w467) -> (value=w452:i32, error out=w470:errorcluster)  [unwired: 4 in]
                "PWM" <- w452
                n204 = Unflatten From JSON(path=string[] ["Imp"], JSON string=w463, type and defaults=w467, error in (no error)=w470) -> (value=w451:i32, error out=w468:errorcluster)  [unwired: 3 in]
                "Tacho" <- w451
                n205 = Unflatten From JSON(path=string[] ["Outputs"], JSON string=w463, type and defaults=w467, error in (no error)=w468) -> (value=w458:i32, error out=w465:errorcluster)  [unwired: 3 in]
                "value" <- w458
                n206 = Number To Boolean Array(number=w458) -> (Boolean array=w457:bool[])
                n207 = Unflatten From JSON(path=string[] ["dP"], JSON string=w463, type and defaults=0.0, error in (no error)=w465) -> (value=w460:dbl)  [unwired: 3 in, 1 out]
                n208 = Index Array(array=w457) -> (element #1=w454:bool, element #2=w453:bool, element #3=w456:bool, element #4=w455:bool)  [unwired: 4 in]
                "GAZ" <- w454
                "Awaria" <- w453
                n209 = Bundle By Name(cluster=w461, "Inputs.PWM"=w452, "Inputs.Tacho"=w451, "Inputs.Gaz"=w454, "Inputs.Awaria"=w453, "Inputs.dP"=w460, "Inputs.Praca"=w456, "Inputs.DKG"=w455) -> (w459:T10)
              }
              frame "OmegaMoc" {
                n210 = Scan From String(format string="%.;%f", input string=w476) -> (output 1=w473:dbl)  [unwired: 3 in, 3 out]
                "MOC" <- w473
                n211 = Bundle By Name(cluster=w475, "Inputs.Power"=w473) -> (w474:T10)
              }
            }
          }
          event "Uruchamia:": Value Change {
            n212 = event-data() -> ("NewVal"=w481:u16)  [unwired: 1 in, 5 out]
            n213 = Unbundle By Name(w480) -> ("Kto-Lista-Num"=w484:i32[])
            n214 = Index Array(array=w484, index=w481) -> (element=w483:i32)
            n215 = Bundle By Name(cluster=w480, "Kto"=w483, "Data.data.Uruchomil"=w483) -> (w479:T10)
          }
          event "Start": Value Change {
            n216 = event-data() -> ()  [unwired: 1 in, 6 out]
            n217 = call <vilib>:"Add State(s) to Queue__JKI_lib_State_Machine.vi"("State(s) in Front (\"\")"="UI: Controls >> ON" ("State(s) at Back (\"\")"), "State(s) in (\"\")"=w488) -> ("States Out"=w489:string)  [unwired: 13 in]
          }
          event "Temat": Value Change {
            n218 = event-data() -> ("NewVal"=w513:u16)  [unwired: 1 in, 5 out]
            n219 = Unbundle By Name(w508) -> ("Tematy-Lista"=w512:string[], "TematyDane"=w511:string[][])
            n220 = call "TematyDane.vi"("Value"=w513, "TematyDane in"=w511, "Tematy-Lista"=w512) -> ("Array"=w505:i32[], "Dane"=w504:string[], "Podtemat"=w507:string, "Temat"=w506:string)  [unwired: 5 in]
            n221 = Index Array(array=w504) -> (element #1=→"SNW":string, element #2=→"SNP":string, element #3=→"Typ Wymiennika":string, element #4=→"Typ Palnika":string)  [unwired: 4 in]
            n222 = Index Array(array=w505) -> (element #1=w499:i32, element #2=w498:i32, element #3=w497:i32, element #4=w496:i32, element #5=w495:i32, element #6=w494:i32)  [unwired: 6 in]
            "Moc Zamowiona" <- w496
            n223 = local write "Zapisane"(FALSE ("Zapisane")) -> ()
            n224 = local write "PWMStart"(w499) -> ()
            n225 = Bundle By Name(cluster=w508, "Temat"=w506, "Data.data.Temat"=w506, "Data.data.Podtemat"=w507, "PWM.start"=w499, "PWM.min"=w498, "PWM.max"=w497, "PWM.moc"=w496, "PWM.min klient"=w495, "PWM.max klient"=w494) -> (w509:T10)
            n226 = local write "PWM Max"(w497) -> ()
            n227 = local write "PWMMin"(w498) -> ()
            n228 = local write "PWM Max Klient"(w495) -> ()
            n229 = local write "PWMMinKlient"(w494) -> ()
          }
          event Panel Close? {
            # "Discard the event because we'll close the front panel ourselves in Macro: Exit"
            # "Close Panel button (pressed) Event\n(this executes Macro: Exit to terminate the VI)"
            n230 = event-data() -> ()  [unwired: 1 in, 1 out]
            n231 = event-data("Discard?"=TRUE) -> ()  [unwired: 1 in, 1 out]
            n232 = call <vilib>:"Add State(s) to Queue__JKI_lib_State_Machine.vi"("State(s) in Front (\"\")"="Macro: Exit", "State(s) in (\"\")"=w520) -> ("States Out"=w519:string)  [unwired: 13 in]
          }
        }
      }
      frame "---------- Core ----------" {
        # "Do not put any code in this frame.\n(it is a separator no-op)"
        n233 = call <vilib>:"Add State(s) to Queue__JKI_lib_State_Machine.vi"("State(s) in (\"\")"=w525) -> ("States Out"=w524:string)  [unwired: 14 in]
      }
      frame Default {
        w536 = 42 items=["No error", "Argument error", "Memory is full", "Out of zone", "End of file", "File already open", "Generic file I/O error", "File not found", "File permission error", "Disk is full", "Duplicate path", "Too many files open", "System feature not enabled", "Resource file not found", "Cannot add resource", "Resource not found", "Image not found", "Image memory error", "Pen does not exist", "Config type invalid", "Config token not found", "Config parse error", "Config memory error", "Bad external code format", "Bad external code offset", "External code not present", "Null window", "Destroy window error", "Null menu", "Print aborted", "Bad print record", "Print driver error", "Windows error during printing", "Memory error during printing", "Print dialog error", "Generic print error", "Invalid device refnum", "Device not found", "Device parameter error", "Device unit error", "Cannot open device", "Device call aborted", "Generic error", "Cancelled by user", "Object ID too low", "Object ID too high", "Object not in heap", "Unknown heap", "Unknown object (invalid DefProc)", "Unknown object (DefProc not in table)", "Message out of range", "Invalid (null) method", "Unknown message", "Manager call not supported", "Bad address", "Network operation in progress", "Network operation timed out", "Connection is busy", "Network attribute not supported", "Network error", "Address in use", "System out of memory", "Connection aborted", "Connection refused", "Not connected", "Already connected", "Connection closed", "Initialization error (interapplication manager)", "Bad occurrence", "Wait on unbound occurrence handler", "Occurrence queue overflow", "Datalog type conflict", "Unused", "Unrecognized type (interapplication manager)", "Memory corrupt", "Failed to make temporary DLL", "Old CIN version", "Drag socket not found", "Failed to load drop-object", "Failed to register OLE object", "Failed to release OLE object", "Format specifier type mismatch", "Unknown format specifier", "Too few format specifiers", "Too many format specifiers", "Scan failed", "Newer CIN version", "Error converting to variant", "Runtime menu error", "Password tampered", "Variant attribute not found", "Incompatible variant data type", "Event data is not available", "Event Store is not present", "Occurrence is not found", "Event Queue is not created", "Event info is not available", "Refnum passed is NULL", "Error retrieving Class GUID", "Error retrieving CoClass GUID", "Error retrieving TypeLib GUID.", "Bad built application magic bytes.", "Specific driver is different from the specific driver associated with the Logical Name.", "There is no session opened to the class driver.", "Max Error", "MAX - Error with config objects", "MAX - Error loading configuration", "MAX - Group not supported"]
        # "Current State"
        # "Do not delete, rename, or modify this frame.\n(this is used to capture unhandled states and typos)"
        # "Handle mistyped state name (developer tool)"
        n234 = Format Into String(format string="Software Exception: Unhandled State \"%s\"." ("message"), error in=w532, w527) -> (resulting string=w535:string, error out=w534:errorcluster)  [unwired: 1 in]
        n235 = call <vilib>:"Error Cluster From Error Code.vi"("show call chain? (False)"=TRUE, "error in (no error)"=w534, "error message (\"\")"=w535, "error code (0)"=w536) -> ("error out"=w533:errorcluster)  [unwired: 5 in]
        n236 = call <vilib>:"Add State(s) to Queue__JKI_lib_State_Machine.vi"("State(s) in (\"\")"=w531) -> ("States Out"=w530:string)  [unwired: 14 in]
      }
      frame "Initialize Core Data" {
        # "Do not delete, rename, or modify this frame.\n(this is used to determine panel behavior on exit)"
        # "originally closed?"
        # "exe?"
        # "If panel starts closed or is an EXE, then close it when we exit"
        n237 = property class="VI"() -> ("Front Panel.Open"=w547:bool)  [unwired: 2 in, 2 out]
        n238 = property class="App"() -> ("App.Kind"=w546:T6)  [unwired: 2 in, 2 out]
        n239 = control-ref of="Current VI Reference"() -> (w540:refnum<vi>)
        n240 = Not(x=w547) -> (.not. x?=w544:bool)
        n241 = Equal?(x=w546, y=T6."Run Time System" ("Application:Kind")) -> (x = y?=w543:bool)
        n242 = Or(x=w544, y=w543) -> (x .or. y?=w541:bool)
        n243 = Bundle By Name(cluster=w542, "Core.Current VI Reference"=w540, "Core.Close Panel on Exit?"=w541, "controls"=w538) -> (w549:T10)
        n244 = call <vilib>:"Add State(s) to Queue__JKI_lib_State_Machine.vi"("State(s) in (\"\")"=w551) -> ("States Out"=w550:string)  [unwired: 14 in]
      }
      frame "Error Handler" {
        # "Unhandled Error -- Display it"
        # "Handle any errors here.\nYou can also output any states to clean-up after errors occur"
        # "Clear error"
        n245 = call <vilib>:"General Error Handler.vi"("error in (no error)"=w554) -> ()  [unwired: 10 in, 5 out]
        n246 = call <vilib>:"Add State(s) to Queue__JKI_lib_State_Machine.vi"("State(s) in Front (\"\")"="/* Post Error States", "State(s) in (\"\")"=w558) -> ("States Out"=w557:string)  [unwired: 13 in]
      }
      frame "Exit" {
        # "Do not put any code in this frame.\n(No errors that occur here will be handled.)"
        n247 = Unregister For Events(event registration refnum=w565, error in=w561) -> (error out=w563:errorcluster)
        n248 = call "disconnect.vi"("error in (no error)"=w563, "Module ID"=w562) -> ("error out"=w564:errorcluster)  [unwired: 9 in]
        n249 = call "Stop Module.vi"("error in (no error)"=w564, "Module ID"=w562) -> ("error out"=w560:errorcluster)  [unwired: 9 in]
        n250 = call <vilib>:"Add State(s) to Queue__JKI_lib_State_Machine.vi"("State(s) in (\"\")"=w569) -> ("States Out"=w568:string)  [unwired: 14 in]
      }
      frame "---------- Data ----------" {
        # "Do not put any code in this frame.\n(It is a separator no-op. You can make a copy of this frame to create a new Data frame)"
        n251 = call <vilib>:"Add State(s) to Queue__JKI_lib_State_Machine.vi"("State(s) in (\"\")"=w574) -> ("States Out"=w573:string)  [unwired: 14 in]
      }
      frame "Data: Initialize" {
        w575 = ""  # Analiza
        w577 = T9 {"Power"=0.0, "PWM"=0, "Tacho"=0, "Gaz"=FALSE, "Awaria"=FALSE, "dP"=0.0, "Praca"=FALSE, "DKG"=FALSE}  # Inputs
        w578 = variant  # Subscriptions
        w579 = variant  # broadcasts
        w580 = 0  # CurrentPWM
        w581 = T11 {" start"=45, "min"=10, "max"=100, "moc"=100, "min klient"=10, "max klient"=100}  # PWM
        w591 = string[][] []  # TematyDane
        w588 = ""  # Temat
        w592 = string[] []  # Tematy-Lista
        w597 = i32[] []  # Kto-Lista-Num
        w593 = u8 0  # Kto
        w596 = string[] []  # Kto-Lista
        w598 = refnum<vi>[] []  # controls
        w599 = T12 {"Current VI Reference"=refnum, "Close Panel on Exit?"=FALSE}  # Core
        # "Data names and types of shift register data are defined by this bundle."
        # "Initialize the shift-register data, here.\n(data names are defined by what you wire into the bundle function)"
        n252 = Insert Into Array(array=w596, new element=w587) -> (w595:string[])  [unwired: 1 in]
        n253 = Insert Into Array(array=w597, new element=w586) -> (w594:i32[])  [unwired: 1 in]
        n254 = Insert Into Array(array=w591, new element=w584) -> (w589:string[][])  [unwired: 2 in]
        n255 = Insert Into Array(array=w592, new element=w585) -> (w590:string[])  [unwired: 1 in]
        n256 = Bundle(w582, "Core"=w599, "controls"=w598, "Kto-Lista"=w595, "Kto-Lista-Num"=w594, "Kto"=w593, "Tematy-Lista"=w590, "TematyDane"=w589, "Temat"=w588, "Data"=T7 {"P"={"max"=0.0, "min"=0.0, "klientmax"=0.0, "klientmin"=0.0}, "CO"={"max"=0.0, "min"=0.0, "klientmax"=0.0, "klientmin"=0.0}, "CO2"={"max"=0.0, "min"=0.0, "klientmax"=0.0, "klientmin"=0.0}, "O2"={"max"=0.0, "min"=0.0, "klientmax"=0.0, "klientmin"=0.0}, "I"={"max"=0.0, "min"=0.0, "klientmax"=0.0, "klientmin"=0.0}, "n"={"max"=0.0, "min"=0.0, "klientmax"=0.0, "klientmin"=0.0}, "pwm"={"klientmax"=0.0, "klientmin"=0.0}, "valve"={"SK"=0.0, "SV"=0.0}, "pLufa100"=0.0, "data"={"Uruchomil"=0.0, "Temat"="", "Podtemat"="", "Uwagi"=""}}, "PWM"=w581, "CurrentPWM"=w580, "broadcasts"=w579, "Subscriptions"=w578, "Inputs"=w577, "Analiza"=w575) -> (w601:T10)  [unwired: 1 in]
        n257 = call <vilib>:"Add State(s) to Queue__JKI_lib_State_Machine.vi"("State(s) in (\"\")"=w603) -> ("States Out"=w602:string)  [unwired: 14 in]
      }
      frame "Data: Cleanup" {
        # "Cleanup any data and references, here.\n(this is called automatically, by the Macro: Exit)"
        n258 = Unbundle By Name(w605) -> ("Core.Current VI Reference"=w608:refnum<vi>)
        n259 = Close Reference(reference=w608, error in (no error)=w607) -> (error out=w606:errorcluster)
        n260 = call <vilib>:"Add State(s) to Queue__JKI_lib_State_Machine.vi"("State(s) in (\"\")"=w610) -> ("States Out"=w609:string)  [unwired: 14 in]
      }
      frame "------MQTT--------" {
        # "Do not put any code in this frame.\n(It is a separator no-op. You can make a copy of this frame to create a new Data frame)"
        n261 = call <vilib>:"Add State(s) to Queue__JKI_lib_State_Machine.vi"("State(s) in (\"\")"=w615) -> ("States Out"=w614:string)  [unwired: 14 in]
      }
      frame "MQTT: Configure" {
        # "Do not put any code in this frame.\n(It is a separator no-op. You can make a copy of this frame to create a new Data frame)"
        n262 = call <vilib>:"Application Directory.vi"() -> ("Application Directory"=w621:path)
        n263 = call "ConfigureMQTT.vi"("error in (no error)"=w623, "base path"=w621, "Module ID"=w624) -> ("error out"=w622:errorcluster, "Subscriptions"=w617:variant, "broadcasts"=w618:variant)  [unwired: 6 in]
        n264 = Bundle By Name(cluster=w620, "broadcasts"=w618, "Subscriptions"=w617) -> (w619:T10)
        n265 = call <vilib>:"Add State(s) to Queue__JKI_lib_State_Machine.vi"("State(s) in (\"\")"=w626) -> ("States Out"=w625:string)  [unwired: 14 in]
      }
      frame "---------- UI ----------" {
        # "Do not put any code in this frame.\n(It is a separator no-op. You can make a copy of this frame to create a new UI frame)"
        n266 = call <vilib>:"Add State(s) to Queue__JKI_lib_State_Machine.vi"("State(s) in (\"\")"=w631) -> ("States Out"=w630:string)  [unwired: 14 in]
      }
      frame "UI: Initialize" {
        # "Initialize the User Interface, here.\n(this is called automatically, by the Macro: Init)"
        n267 = call <vilib>:"Add State(s) to Queue__JKI_lib_State_Machine.vi"("State(s) in (\"\")"=w636) -> ("States Out"=w635:string)  [unwired: 14 in]
      }
      frame "UI: Controls" {
        # "Initialize the User Interface, here.\n(this is called automatically, by the Macro: Init)"
        n268 = Equal?(x=w637, y="ON") -> (x = y?=w640:bool)
        n269 = Not(x=w640) -> (.not. x?=w641:bool)
        n270 = Unbundle By Name(w648) -> ("controls"=w649:refnum<vi>[])
        n271 = Select(t=T5."Enabled" ("Disabled"), s=w641, f=T5."Disabled and Grayed Out" ("Disabled")) -> (s? t:f=w642:T5)
        n272 = Select(t=T5."Enabled" ("Disabled"), s=w640, f=T5."Disabled and Grayed Out" ("Disabled")) -> (s? t:f=w645:T5)
        n273 = for {
          tunnel: w649 -> [w654] mode=indexing
          tunnel: w645 -> [w653]
          n274 = property class="Ctl"(reference=w654, "DisabledEnum"=w653) -> ()  [unwired: 1 in, 2 out]
        }
        n275 = property on="Start" class="Bool"("DisabledEnum"=w642) -> ()  [unwired: 2 in, 2 out]
        n276 = call <vilib>:"Add State(s) to Queue__JKI_lib_State_Machine.vi"("State(s) in (\"\")"=w652) -> ("States Out"=w651:string)  [unwired: 14 in]
      }
      frame "UI: Cursor Set" {
        # "Argument"
        # "Set and Unset Cursor Busy.\n(Usage: \"UI: Cursor Set >> Busy|Idle\")"
        n277 = case shown="\"Idle\", Default" w656 {
          tunnel: w658 -> [w663 w665]
          tunnel: [w662 w664] -> w657
          frame "Idle", Default {
            n278 = call <vilib>:"Unset Busy.vi"("error in (no error)"=w663) -> ("error out"=w662:errorcluster)  [unwired: 10 in]
          }
          frame "Busy" {
            n279 = call <vilib>:"Set Busy.vi"("error in (no error)"=w665) -> ("error out"=w664:errorcluster)  [unwired: 9 in, 1 out]
          }
        }
        n280 = call <vilib>:"Add State(s) to Queue__JKI_lib_State_Machine.vi"("State(s) in (\"\")"=w661) -> ("States Out"=w660:string)  [unwired: 14 in]
      }
      frame "UI: Front Panel State" {
        # "Argument"
        # "Set Front Panel Open or Closed\n(Usage: \"UI: Front Panel State >> Open|Close\")"
        n281 = Unbundle By Name(w669) -> ("Core.Current VI Reference"=w668:refnum<vi>)
        n282 = case shown="\"Open\", Default" w667 {
          tunnel: w671 -> [w677 w690]
          tunnel: [w679 w691] -> w670
          tunnel: w668 -> [w678 w688]
          frame "Open", Default {
            n283 = property class="VI"(reference=w678, error in=w677) -> (reference out=w675:refnum<vi>, error out=w676:errorcluster, "Front Panel.Open"=w674:bool)
            n284 = case shown="True" w674 {
              tunnel: [w682 w685] -> w679
              tunnel: w676 -> [w681 w685]
              tunnel: w675 -> [w680 _]
              frame False {
                n285 = invoke class="VI" method="FP.Open"(reference=w680, error in=w681, "Activate"=TRUE, "State"=T8."Standard") -> (error out=w682:errorcluster)  [unwired: 1 in, 4 out]
              }
              frame True {
              }
            }
          }
          frame "Close" {
            n286 = property class="VI"(reference=w688, error in=w690) -> (reference out=w687:refnum<vi>, error out=w689:errorcluster, "Front Panel.Open"=w686:bool)
            n287 = case shown="True" w686 {
              tunnel: [w692 w695] -> w691
              tunnel: w689 -> [w692 w694]
              tunnel: w687 -> [_ w693]
              frame False {
              }
              frame True {
                n288 = invoke class="VI" method="FP.Close"(reference=w693, error in=w694) -> (error out=w695:errorcluster)  [unwired: 1 in, 2 out]
              }
            }
          }
        }
        n289 = call <vilib>:"Add State(s) to Queue__JKI_lib_State_Machine.vi"("State(s) in (\"\")"=w673) -> ("States Out"=w672:string)  [unwired: 14 in]
      }
      frame "---------- Macro ----------" {
        # "Do not put any code in this frame.\n(It is a separator no-op. You can make a copy of this frame to create a new Macro frame)"
        n290 = call <vilib>:"Add State(s) to Queue__JKI_lib_State_Machine.vi"("State(s) in (\"\")"=w700) -> ("States Out"=w699:string)  [unwired: 14 in]
      }
      frame "Macro: Initialize" {
        w702 = "Data: Initialize\nInitialize Core Data\nMQTT: Configure\nUI: Initialize\nUI: Front Panel State >> Open\nUI: Controls >> OFF"  # Data: Initialize Initialize Core Data MQTT: Configure UI: Initialize UI: Front Panel State >> Open UI: Controls >> OFF
        # "Initialization Macro\n(This is called once, when the VI starts)"
        n291 = call <vilib>:"Add State(s) to Queue__JKI_lib_State_Machine.vi"("State(s) in Front (\"\")"=w702, "State(s) in (\"\")"=w706) -> ("States Out"=w705:string)  [unwired: 13 in]
      }
      frame "Macro: Exit" {
        # "Exit Macro\n(This is called once, when the VI exits)"
        n292 = Unbundle By Name(w714) -> ("Core.Close Panel on Exit?"=w713:bool)
        n293 = Select(t="UI: Front Panel State >> Close", s=w713, f="") -> (s? t:f=w710:string)
        n294 = call <vilib>:"Add State(s) to Queue__JKI_lib_State_Machine.vi"("State(s) in (\"\")"=w710, "State(s) at Back (\"\")"="Data: Cleanup\nExit") -> ("States Out"=w708:string)  [unwired: 13 in]
        n295 = call <vilib>:"Add State(s) to Queue__JKI_lib_State_Machine.vi"("State(s) in Front (\"\")"=w708, "State(s) in (\"\")"=w717) -> ("States Out"=w716:string)  [unwired: 13 in]
      }
      frame "---------- New Category ----------" {
        # "Template Separator\n(You can make a copy of, or modify, this frame)"
        n296 = call <vilib>:"Add State(s) to Queue__JKI_lib_State_Machine.vi"("State(s) in (\"\")"=w722) -> ("States Out"=w721:string)  [unwired: 14 in]
      }
      frame "New Category: 1" {
        # "Your code here.\n(You can make a copy of, or modify, this frame)"
        n297 = call <vilib>:"Add State(s) to Queue__JKI_lib_State_Machine.vi"("State(s) in (\"\")"=w727) -> ("States Out"=w726:string)  [unwired: 14 in]
      }
      frame "New Category: 2" {
        # "Your code here.\n(You can make a copy of, or modify, this frame)"
        n298 = call <vilib>:"Add State(s) to Queue__JKI_lib_State_Machine.vi"("State(s) in (\"\")"=w732) -> ("States Out"=w731:string)  [unwired: 14 in]
      }
    }
  }
